vi "Read SV.vi"(8 "error in (no error)":errorcluster, 10 "Data":dbl[](array[numeric]), 11 "Read Refs by Type":T1) -> (0 "error out":errorcluster, 2 "Data Out":dbl[](array[numeric]))   [LabVIEW 2016, in "Shared Variable Interface.lvlib"]
uses:
  Shared Variable Interface.lvlib
  DataTypes/DBL.lvlib
  DataTypes/Bool.lvlib
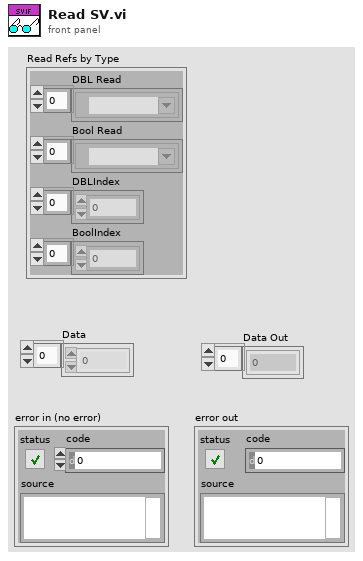
[diagram p1: front panel]
types:
  T1 = cluster{"DBL Read":refnum<k21>[], "Bool Read":refnum<k21>[], "DBLIndex":i32[], "BoolIndex":i32[]}
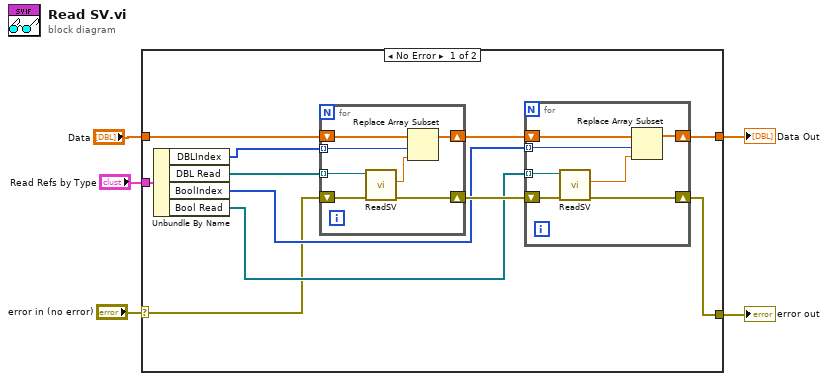
[diagram p0: block diagram]
diagram:
  n1 = case shown="No Error" "error in (no error)" {
    selector: "error in (no error)" -> [w6 w32]
    tunnel: [w15 w32] -> w5
    tunnel: "Data" -> [w14 w31]
    tunnel: [w10 w31] -> w3
    tunnel: "Read Refs by Type" -> [w7 _]
    frame No Error {
      n2 = Unbundle By Name(w7) -> ("DBLIndex"=w8:i32[], "DBL Read"=w13:refnum<k21>[], "BoolIndex"=w9:i32[], "Bool Read"=w12:refnum<k21>[])
      n3 = for {
        shift-right: [w29] -> w16
        shift-left: w6 -> [w30]
        shift-right: [w27] -> w11
        shift-left: w14 -> [w26]
        tunnel: w13 -> [w25] mode=indexing
        tunnel: w8 -> [w24] mode=indexing
        n4 = call "ReadSV.vi"("error in (no error)"=w30, "shared variable refnum"=w25) -> ("error out"=w29:errorcluster, "DBL Data"=w28:dbl)  [unwired: 8 in]
        n5 = Replace Array Subset(array=w26, new element=w28, index=w24) -> (w27:dbl[])
      }
      n6 = for {
        tunnel: w12 -> [w21] mode=indexing
        shift-right: [w22] -> w15
        shift-left: w16 -> [w23]
        shift-right: [w19] -> w10
        shift-left: w11 -> [w20]
        tunnel: w9 -> [w17] mode=indexing
        n7 = call "ReadSV.vi"("error in (no error)"=w23, "shared variable refnum in"=w21) -> ("error out"=w22:errorcluster, "DBL Data"=w18:dbl)  [unwired: 8 in]
        n8 = Replace Array Subset(array=w20, new element=w18, index=w17) -> (w19:dbl[])
      }
    }
    frame Error {
    }
  }
  "error out" <- w5
  "Data Out" <- w3
